vi "Write Reader.vi"(8 "Error In":errorcluster, 10 "Reader":refnum<class "Reader.lvclass">, 11 "Lexer In":refnum<class "Lexer.lvclass">) -> (0 "Error Out":errorcluster, 3 "Lexer Out":refnum<class "Lexer.lvclass">)   [LabVIEW 2018, in "Toolkit.lvlib" / "Lexer.lvclass"]
uses:
  Lexer.lvclass
  Readers/Reader/Reader.lvclass
  Lexer.lvclass/Lexer.ctl
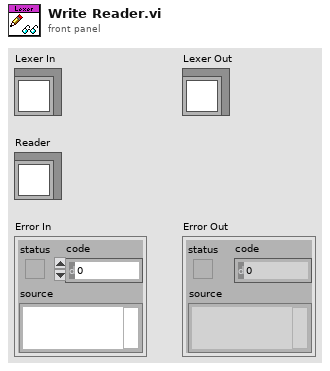
[diagram p1: front panel]
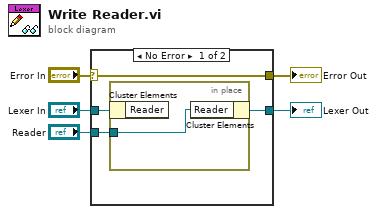
[diagram p0: block diagram]
diagram:
  n1 = case shown="No Error" "Error In" {
    selector: "Error In" -> [w9 w11]
    tunnel: [w9 w11] -> w4
    tunnel: [w7 w12] -> w2
    tunnel: "Lexer In" -> [w8 w12]
    tunnel: "Reader" -> [w6 _]
    frame No Error {
      n2 = in-place {
        in-place-border: w6 -> [w10]
        n3 = in-place-cluster #1(w8) -> ()  [unwired: 1 out]
        n4 = in-place-cluster #1("Reader"=w10) -> (w7:refnum<class "Lexer.lvclass">)
      }
    }
    frame Error {
    }
  }
  "Error Out" <- w4
  "Lexer Out" <- w2
